vi "Standby Power Check Final Conditions.vi"(5 "Standby Power In":T1, 7 "Power":T2={"Yokogawa"={"WT210"={"Sample Rate (1: 0.25s)"=0, "A Range (12: 20A)"=0, "V Range (6: 600V)"=0, "Power VISA Yokogawa WT210"=""}, "WT500"={"Power VISA Yokogawa WT500"="", "V Range (8: 1000V)"=0, "I Range (7: 40A)"=0, "Update Rate (3: 500ms)"=0}, "WT310_2"={"Sample Rate (1: 0.25s)"=1, "A Range (12: 20A)"=11, "V Range (6: 600V)"=4, "Power VISA Yokogawa WT310_2"=""}, "WT310_3"={"Sample Rate (1: 0.25s)"=1, "A Range (12: 20A)"=11, "V Range (6: 600V)"=4, "Power VISA Yokogawa WT310_3"=""}}, "Aplus"={"Aplus IP Address"="", "Remote Port"=0, "Instrument"="", "Instr Driver Revision"=""}, "Power Limits"={"Crest Factor"={"Upper Limit"=0.0, "Lower Limit"=0.0}, "Harmonic Content"={"Uthd"=0.0}, "Voltage"={"% Error"=0.0}, "Stability"={"<1 Watt "={"Wattage"=0.0, "Slope (mW/H)"=0.0}, ">1 Watt"={"1%Power/Hour"=0.0}}}, "Nominal Voltage"=0, "Time Limit (s)"=0.0, "Power Variation Limit (%)"=0.0, "Power Supply"={"Chroma 61605"="", "Use Chroma?"=FALSE}} {"Yokogawa"."WT310_3"."V Range (6: 600V)" items=["Auto", "15V", "30V", "60V", "150V", "300V", "600V"]; "Yokogawa"."WT310_3"."A Range (12: 20A)" items=["Auto", "5mA", "10mA", "20mA", "50mA", "100mA", "200mA", "0.5A", "1A", "2A", "5A", "10A", "20A", "50mV", "100mV", "200mV", "2.5V", "5V", "10V"]; "Yokogawa"."WT310_3"."Sample Rate (1: 0.25s)" items=["0.1s", "0.25s", "0.5s", "1s", "2s", "5s"]; "Yokogawa"."WT310_2"."V Range (6: 600V)" items=["Auto", "15V", "30V", "60V", "150V", "300V", "600V"]; "Yokogawa"."WT310_2"."A Range (12: 20A)" items=["Auto", "5mA", "10mA", "20mA", "50mA", "100mA", "200mA", "0.5A", "1A", "2A", "5A", "10A", "20A", "50mV", "100mV", "200mV", "2.5V", "5V", "10V"]; "Yokogawa"."WT310_2"."Sample Rate (1: 0.25s)" items=["0.1s", "0.25s", "0.5s", "1s", "2s", "5s"]; "Yokogawa"."WT500"."Update Rate (3: 500ms)" items=["-", "100ms", "200ms", "500ms", "1s", "2s", "5s"]; "Yokogawa"."WT500"."I Range (7: 40A)" items=["AUTO", "500 mA", "1 A", "2 A", "5 A", "10 A", "20 A", "40 A", "S-AUTO", "50 mV", "100 mV", "200 mV", "500 mV", "1 V", "2 V", "5 V", "10 V", "250 mA", "500 mA", "1 A", "2.5 A", "5 A", "10 A", "20 A", "25 mV", "50 mV", "100 mV", "250 mV", "500 mV", "1 V", "2.5 V", "5 V"]; "Yokogawa"."WT500"."V Range (8: 1000V)" items=["AUTO", "15", "30", "60", "100", "150", "300", "600", "1000", "7.5", "15", "30", "50", "75", "150", "300", "500"]; "Yokogawa"."WT210"."V Range (6: 600V)" items=["Auto", "15V", "30V", "60V", "150V", "300V", "600V"]; "Yokogawa"."WT210"."A Range (12: 20A)" items=["Auto", "5mA", "10mA", "20mA", "50mA", "100mA", "200mA", "0.5A", "1A", "2A", "5A", "10A", "20A", "50mV", "100mV", "200mV", "2.5V", "5V", "10V"]; "Yokogawa"."WT210"."Sample Rate (1: 0.25s)" items=["0.1s", "0.25s", "0.5s", "1s", "2s", "5s"]}, 8 "Error In":errorcluster, 11 "Slope (mW/hr)":dbl) -> (0 "Error Out":errorcluster, 2 "Test Complete":bool, 3 "Standby Power Out":T1)   [LabVIEW 2018]
uses:
  Type Definitions/UTILITY Power Inputs Control.ctl
  Type Definitions/Standby Power Main Data.ctl
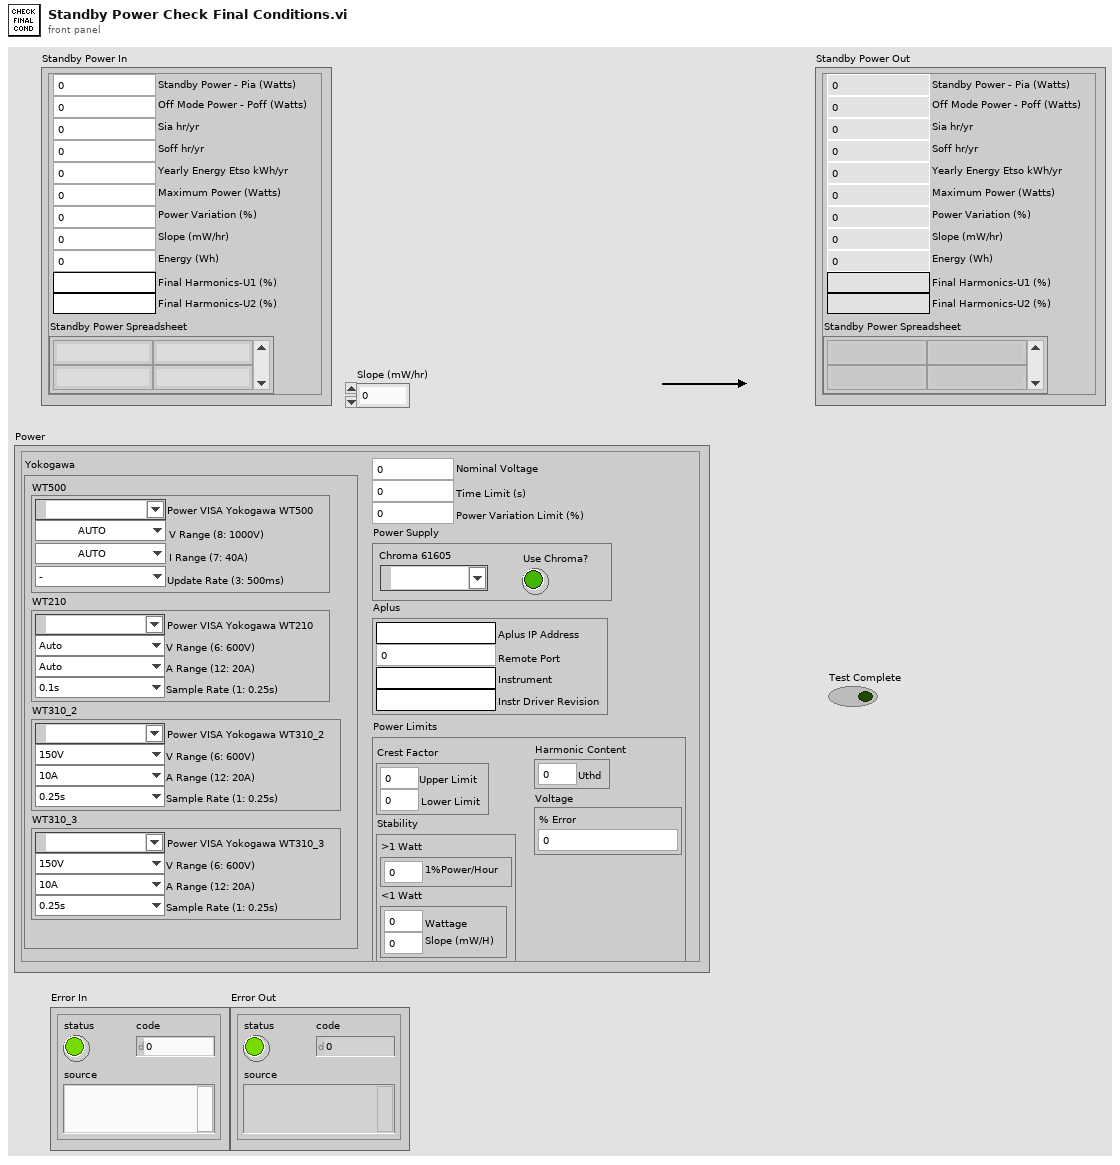
[diagram p1: front panel]
types:
  T1 = typedef "Standby Power Main Data.ctl" = cluster{"Standby Power Spreadsheet":string[][], "Standby Power - Pia (Watts)":dbl, "Off Mode Power - Poff (Watts)":dbl, "Sia hr/yr":dbl, "Soff hr/yr":dbl, "Yearly Energy Etso kWh/yr":dbl, "Maximum Power (Watts)":dbl, "Power Variation (%)":dbl, "Slope (mW/hr)":dbl, "Final Harmonics-U1 (%)":string, "Final Harmonics-U2 (%)":string, "Energy (Wh)":dbl}
  T2 = typedef "UTILITY Power Inputs Control.ctl" = cluster{"Yokogawa":cluster{"WT210":cluster{"Sample Rate (1: 0.25s)":i32, "A Range (12: 20A)":i32, "V Range (6: 600V)":i32, "Power VISA Yokogawa WT210":refnum<visa-resource-name>}, "WT500":cluster{"Power VISA Yokogawa WT500":refnum<visa-resource-name>, "V Range (8: 1000V)":i32, "I Range (7: 40A)":i32, "Update Rate (3: 500ms)":i32}, "WT310_2":cluster{"Sample Rate (1: 0.25s)":i32, "A Range (12: 20A)":i32, "V Range (6: 600V)":i32, "Power VISA Yokogawa WT310_2":refnum<visa-resource-name>}, "WT310_3":cluster{"Sample Rate (1: 0.25s)":i32, "A Range (12: 20A)":i32, "V Range (6: 600V)":i32, "Power VISA Yokogawa WT310_3":refnum<visa-resource-name>}}, "Aplus":cluster{"Aplus IP Address":string, "Remote Port":i32, "Instrument":string, "Instr Driver Revision":string}, "Power Limits":cluster{"Crest Factor":cluster{"Upper Limit":dbl, "Lower Limit":dbl}, "Harmonic Content":cluster{"Uthd":dbl}, "Voltage":cluster{"% Error":dbl}, "Stability":cluster{"<1 Watt ":cluster{"Wattage":dbl, "Slope (mW/H)":dbl}, ">1 Watt":cluster{"1%Power/Hour":dbl}}}, "Nominal Voltage":i32, "Time Limit (s)":dbl, "Power Variation Limit (%)":dbl, "Power Supply":cluster{"Chroma 61605":refnum<visa-resource-name>, "Use Chroma?":bool}}
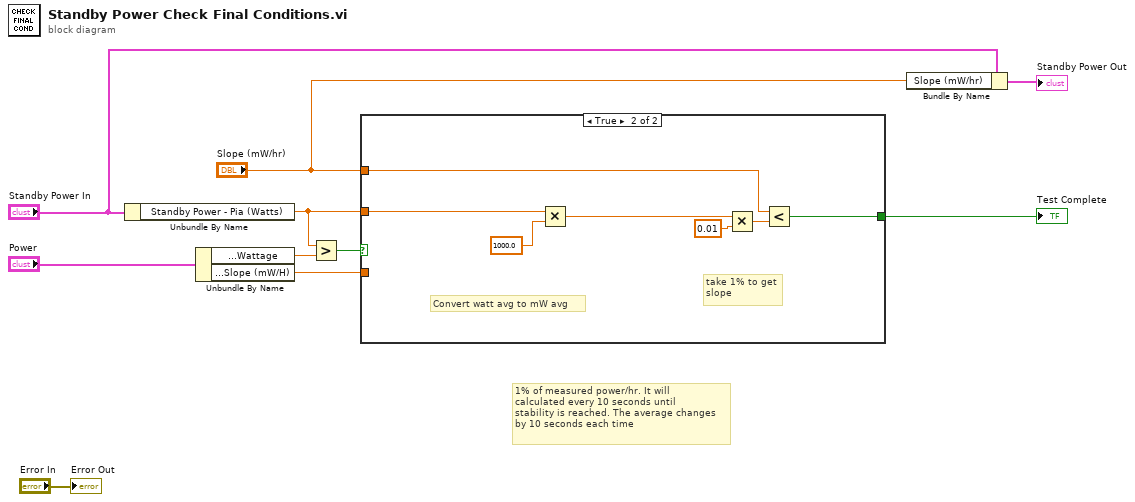
[diagram p0: block diagram]
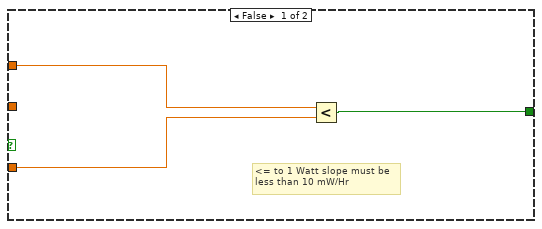
[diagram p2: hidden frame]
diagram:
  # "1% of measured power/hr. It will\ncalculated every 10 seconds until \nstability is reached. The average changes\nby 10 seconds each time"
  n1 = Unbundle By Name("Standby Power In") -> ("Standby Power - Pia (Watts)"=w7:dbl)
  n2 = Unbundle By Name("Power") -> ("Power Limits.Stability.<1 Watt.Wattage"=w9:dbl, "Power Limits.Stability.<1 Watt.Slope (mW/H)"=w10:dbl)
  n3 = Greater?(x=w7, y=w9) -> (0:w6:bool)
  n4 = case shown="True" w6 {
    tunnel: "Slope (mW/hr)" -> [w11 w19]
    tunnel: [w13 w17] -> w5
    tunnel: w10 -> [w12 _]
    tunnel: w7 -> [_ w15]
    frame False {
      # "<= to 1 Watt slope must be\nless than 10 mW/Hr"
      n5 = Less?(x=w11, y=w12) -> (x < y?=w13:bool)
    }
    frame True {
      # "take 1% to get\nslope"
      # "Convert watt avg to mW avg"
      n6 = Multiply(x=w15, y=1000.0) -> (x*y=w14:dbl)
      n7 = Multiply(x=w14, y=0.01) -> (x*y=w18:dbl)
      n8 = Less?(x=w19, y=w18) -> (x < y?=w17:bool)
    }
  }
  "Test Complete" <- w5
  n9 = Bundle By Name(cluster="Standby Power In", "Slope (mW/hr)"="Slope (mW/hr)") -> (→"Standby Power Out":T1)
  "Error Out" <- "Error In"
